vi "Add Plugin Status Sections.vi"(8 "error in (no error)":errorcluster, 11 "Item Ref in":T1 format="%.0x") -> (0 "error out":errorcluster, 3 "Item Ref out":T1 format="%.0x")   [LabVIEW 2017, in "DSF System Explorer.lvlib"]
uses:
  DSF System Explorer.lvlib
  <vilib>/NI Veristand/Custom Device API/Custom Device Item Ref.ctl
  Shared/Plugin Page GUID.vi
  Shared/Group Page GUID.vi
  Shared/Transfer Page GUID.vi
  Shared/DSF Shared.lvlib
  <vilib>/NI Veristand/Custom Device API/Custom Device API.lvlib
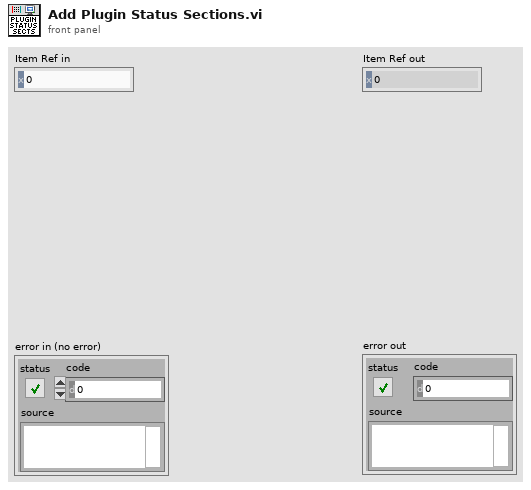
[diagram p1: front panel]
types:
  T1 = typedef "Custom Device API.lvlib/Custom Device Item Ref.ctl" = u64
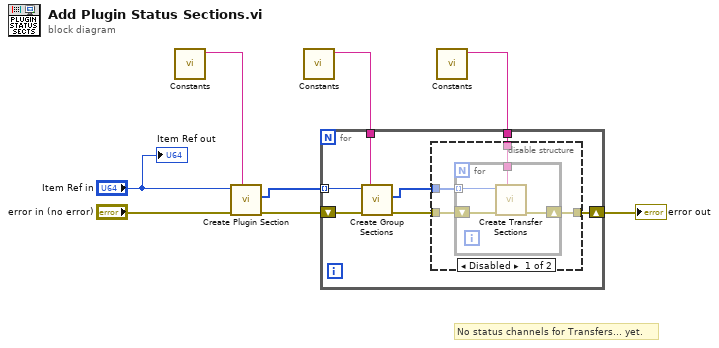
[diagram p0: block diagram]
diagram:
  # "No status channels for Transfers... yet."
  n1 = call-poly "Constants.vi"() -> ("Plugin GUID"=w3:string)  [unwired: 11 in]
  n2 = call "Create Plugin Section.vi"("GUID (Default Section)"=w3, "error in (no error)"="error in (no error)", "Item Ref in"="Item Ref in") -> ("error out"=w7:errorcluster, "Plugin Section refs"=w6:T1[])  [unwired: 6 in, 1 out]
  n3 = call-poly "Constants.vi"() -> ("Group GUID"=w2:string)  [unwired: 11 in]
  n4 = call-poly "Constants.vi"() -> ("Transfer GUID"=w1:string)  [unwired: 11 in]
  n5 = for {
    shift-right: [w11] -> w4
    shift-left: w7 -> [w15]
    tunnel: w6 -> [w14] mode=indexing
    tunnel: w2 -> [w10]
    tunnel: w1 -> [w9]
    n6 = call "Create Group Sections.vi"("GUID (Default Section)"=w10, "error in (no error)"=w15, "Item Ref in"=w14) -> ("error out"=w13:errorcluster, "Group Section refs"=w12:T1[])  [unwired: 6 in, 1 out]
    n7 = disable-structure shown="Disabled" {
      disable-tunnel: w13 -> [w19 w24]
      disable-tunnel: w12 -> [w18 _]
      disable-tunnel: [w17 w24] -> w11
      disable-tunnel: w9 -> [w16 _]
      frame Disabled {
        n8 = for {
          shift-right: [w21] -> w17
          shift-left: w19 -> [w23]
          tunnel: w18 -> [w22] mode=indexing
          tunnel: w16 -> [w20]
          n9 = call "Create Transfer Sections.vi"("GUID (Default Section)"=w20, "error in (no error)"=w23, "Item Ref in"=w22) -> ("error out"=w21:errorcluster)  [unwired: 6 in, 2 out]
        }
      }
      frame Enabled {
      }
    }
  }
  "error out" <- w4
  "Item Ref out" <- "Item Ref in"
